vi "Save_to_DB_subVi.vi"(8 "error in (no error)":errorcluster, 9 "PMS_Data":T1, 10 "Wybranie tabeli z bazy danych":string, 11 "Wybranie bazy danych - plik .UDL":path) -> (0 "error out":errorcluster)   [LabVIEW 2019]
doc: "This VI provides data to be saved to DB. As input we have path to database file, table name, DATA that we use, error in. As output we have error out."
uses:
  Type Definitions/PMS_Data.ctl
  <vilib>/addons/database/Connection.llb/DB Tools Open Connec (Path).vi
  <vilib>/addons/database/NI_Database_API.lvlib
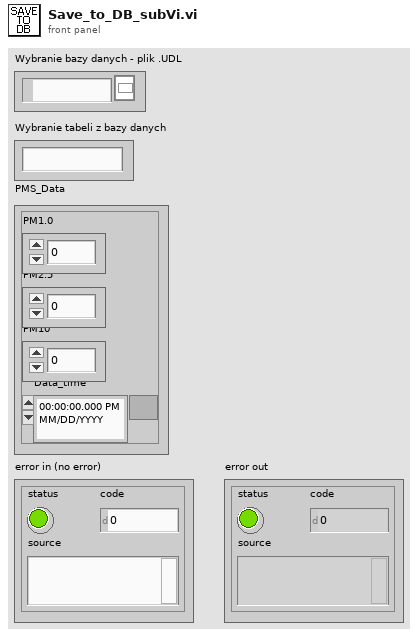
[diagram p1: front panel]
types:
  T1 = typedef "PMS_Data.ctl" = cluster{"PM1.0":i32, "PM2.5":i32, "PM10":i32, "Data_time":timestamp}
  T2 = typedef "NI_Database_API.lvlib/Conn ObjectReference.ctl" = refnum<k1>
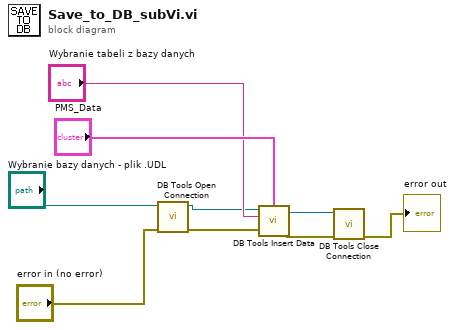
[diagram p0: block diagram]
diagram:
  n1 = call-poly <vilib>:"DB Tools Open Connection.vi"("error in (no error)"="error in (no error)", "connection information"="Wybranie bazy danych - plik .UDL") -> ("error out"=w3:errorcluster, "connection reference"=w2:T2)  [unwired: 6 in]
  n2 = call <vilib>:"DB Tools Insert Data.vi"("data"="PMS_Data", "error in (no error)"=w3, "table"="Wybranie tabeli z bazy danych", "connection reference"=w2) -> ("error out"=w5:errorcluster, "connection reference out"=w4:T2)  [unwired: 6 in]
  n3 = call <vilib>:"DB Tools Close Connection.vi"("error in (no error)"=w5, "connection reference"=w4) -> ("error out"=→"error out":errorcluster)  [unwired: 5 in]
